vi "Get Selected Pattern.vi"(8 "error in (no error)":errorcluster, 10 "Listbox Index":i32, 11 "ListBox in":refnum<vi>) -> (0 "error out":errorcluster, 2 "Pattern Index":i32, 3 "Type":string)   [LabVIEW 2013]
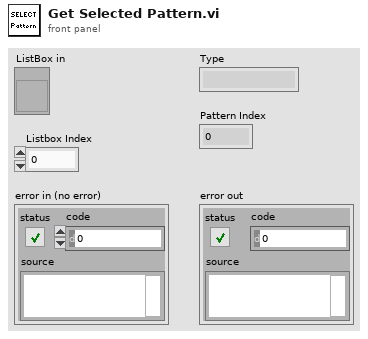
[diagram p1: front panel]
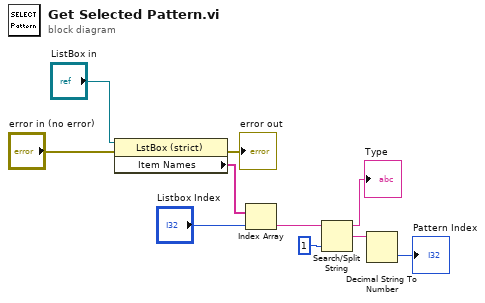
[diagram p0: block diagram]
diagram:
  n1 = property class="LstBox (strict)"(reference="ListBox in", error in="error in (no error)") -> (error out=→"error out":errorcluster, "Item Names"=w2:string[])  [unwired: 1 out]
  n2 = Index Array(array=w2, index="Listbox Index") -> (element=w7:string)
  n3 = Search/Split String(string=w7, offset (0)=1) -> (substring before match=→"Type":string, match + rest of string=w9:string)  [unwired: 1 in, 1 out]
  n4 = Decimal String To Number(string=w9) -> (number=→"Pattern Index":i32)  [unwired: 2 in, 1 out]
